vi "Compute Histogram Halves Standard Deviations.vi"(5 "x 2":dbl, 7 "x 1":dbl, 8 "Error In":errorcluster, 10 "Y Array":dbl[](array[numeric]), 11 "X Array":dbl[](array[numeric])) -> (0 "Error Out":errorcluster, 2 "SDV 2":dbl, 3 "SDV 1":dbl)   [LabVIEW 2019]
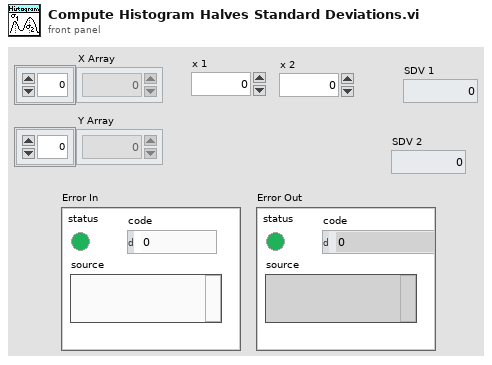
[diagram p1: front panel]
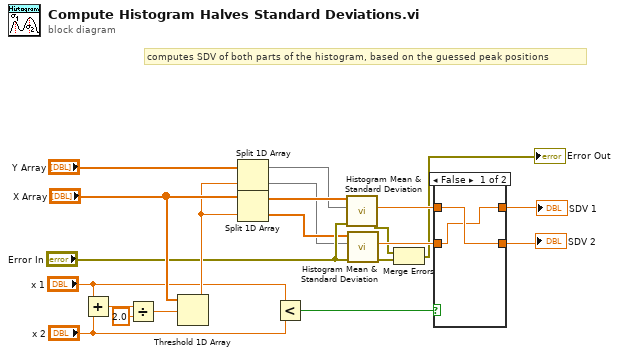
[diagram p0: block diagram]
diagram:
  # "computes SDV of both parts of the histogram, based on the guessed peak positions"
  n1 = Add(x="x 1", y="x 2") -> (x+y=w21:dbl)
  n2 = Divide(x=w21, y=2.0) -> (x/y=w19:dbl)
  n3 = Threshold 1D Array(2:w19, 3:"X Array") -> (0:w16:dbl)  [unwired: 1 in]
  n4 = Split 1D Array(array="Y Array", index=w16) -> (first subarray=w14:dbl[], second subarray=w1:dbl[])
  n5 = Split 1D Array(array="X Array", index=w16) -> (first subarray=w15:dbl[], second subarray=w2:dbl[])
  n6 = Less?(x="x 1", y="x 2") -> (x < y?=w10:bool)
  n7 = call "Histogram Mean & Standard Deviation.vi"("Error In"="Error In", "Histogram"=w14, "Values"=w15) -> ("Error Out"=w4:errorcluster, "Standard Deviation"=w9:dbl)  [unwired: 5 in, 2 out]
  n8 = call "Histogram Mean & Standard Deviation.vi"("Error In"="Error In", "Histogram"=w1, "Values"=w2) -> ("Error Out"=w5:errorcluster, "Standard Deviation"=w7:dbl)  [unwired: 5 in, 2 out]
  n9 = Merge Errors(w4, w5) -> (→"Error Out":errorcluster)
  n10 = case shown="False" w10 {
    tunnel: w9 -> [w23 w25]
    tunnel: [w22 w25] -> w8
    tunnel: w7 -> [w22 w24]
    tunnel: [w23 w24] -> w6
    frame False {
    }
    frame True {
    }
  }
  "SDV 2" <- w6
  "SDV 1" <- w8
